vi "local Variables.vi"() -> ()   [LabVIEW 2024]
panel:
  out "x":dbl
  out "y 3":bool
  out "y 2":dbl
  out "y":bool
  in  "D":dbl
  in  "C":dbl
  in  "B":bool
  in  "A":bool
  in  "stop 2":bool
  in  "stop":bool
  # "Overview:\nIn this VI, local Variables usage is used. \nValues are given to the local variables and are used in the loops."
  # "s"
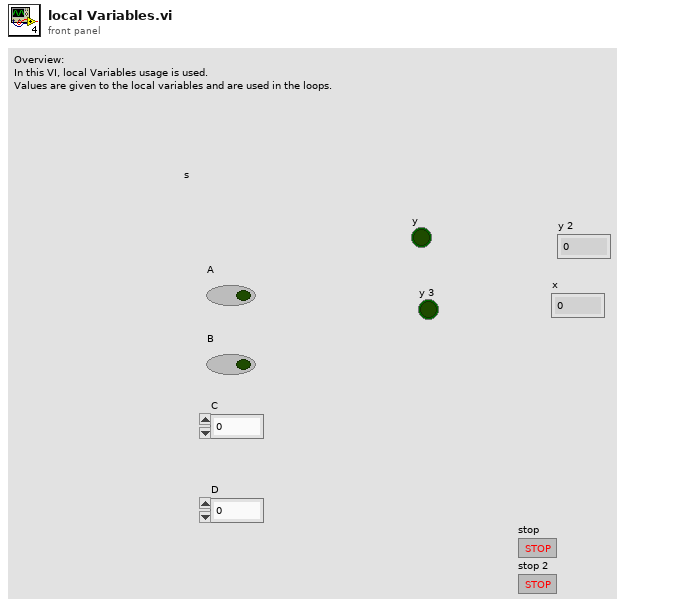
[diagram p1: front panel]
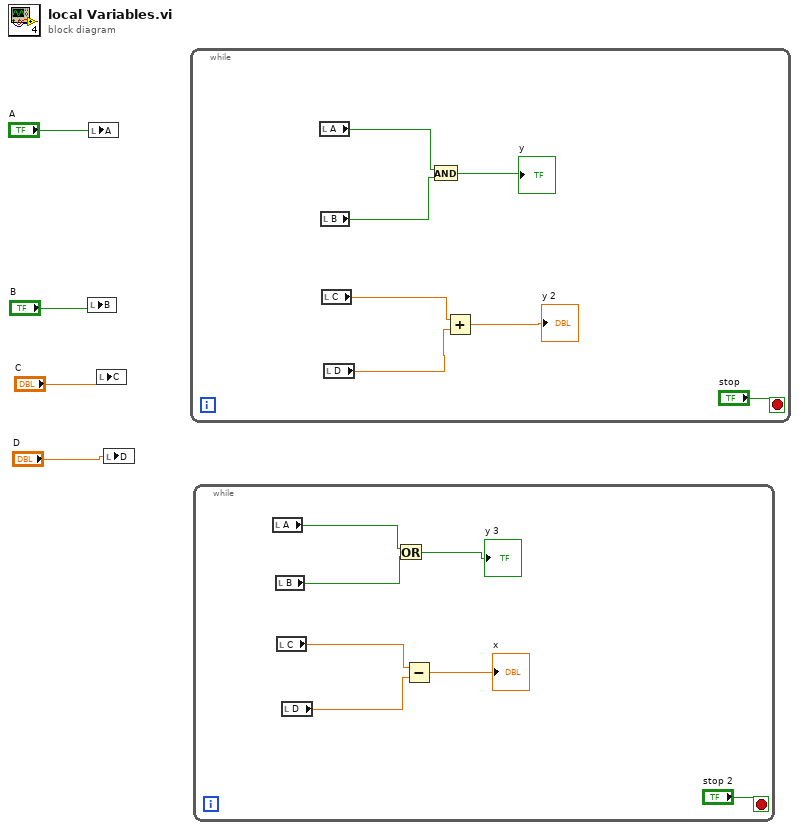
[diagram p0: block diagram]
diagram:
  n1 = local write "B"("B") -> ()
  n2 = local write "A"("A") -> ()
  n3 = local write "C"("C") -> ()
  n4 = local write "D"("D") -> ()
  n5 = while {
    stop <- "stop" stop-if-true
    n6 = local read "A"() -> (w9:bool)
    n7 = local read "B"() -> (w8:bool)
    n8 = local read "C"() -> (w6:dbl)
    n9 = local read "D"() -> (w5:dbl)
    n10 = And(x=w9, y=w8) -> (x .and. y?=→"y":bool)
    n11 = Add(x=w6, y=w5) -> (x+y=→"y 2":dbl)
  }
  n12 = while {
    stop <- "stop 2" stop-if-true
    n13 = local read "A"() -> (w16:bool)
    n14 = local read "B"() -> (w15:bool)
    n15 = local read "C"() -> (w14:dbl)
    n16 = local read "D"() -> (w13:dbl)
    n17 = Or(x=w16, y=w15) -> (x .or. y?=→"y 3":bool)
    n18 = Subtract(x=w14, y=w13) -> (x-y=→"x":dbl)
  }
